vi "Plot Key Down.vi"(7 "Loop data in":T3={"TitleCollapse"=refnum, "MouseDownState"=enum."Idle", "RightClickCache"={"Mod"={"Ctrl"=FALSE, "Shift"=FALSE}, "CoordsStart"={"Horizontal"=0, "Vertical"=0}, "CoordsEnd"={"Horizontal"=0, "Vertical"=0}, "PlotAreaBounds"={"Left"=10, "Top"=10, "Right"=0, "Bottom"=0}, "slice"=[]}, "ZoomCache"={"SuppressedPlots"=[], "LeftAxis"={"NeedsRevert?"=FALSE, "Scale Fit"=0, "Range"={"Minimum"=0.0, "Maximum"=0.0, "Increment"=0.0, "Minor Increment"=0.0, "Start"=0.0}}, "RightAxis"={"NeedsRevert?"=FALSE, "Scale Fit"=0, "Range"={"Minimum"=0.0, "Maximum"=0.0, "Increment"=0.0, "Minor Increment"=0.0, "Start"=0.0}}, "Mod"={"Shift"=FALSE}}, "UpdateTime"=0.0, "keyboard"=refnum, "visible?"=FALSE}, 8 "error in (no error)":errorcluster, 9 "PlatMods":T1, 10 "VKey":T2, 11 "Refs":T14) -> (0 "error out":errorcluster, 3 "Update plot?":bool, 5 "Loop data out":T3={"TitleCollapse"=refnum, "MouseDownState"=enum."Idle", "RightClickCache"={"Mod"={"Ctrl"=FALSE, "Shift"=FALSE}, "CoordsStart"={"Horizontal"=0, "Vertical"=0}, "CoordsEnd"={"Horizontal"=0, "Vertical"=0}, "PlotAreaBounds"={"Left"=10, "Top"=10, "Right"=0, "Bottom"=0}, "slice"=[]}, "ZoomCache"={"SuppressedPlots"=[], "LeftAxis"={"NeedsRevert?"=FALSE, "Scale Fit"=0, "Range"={"Minimum"=0.0, "Maximum"=0.0, "Increment"=0.0, "Minor Increment"=0.0, "Start"=0.0}}, "RightAxis"={"NeedsRevert?"=FALSE, "Scale Fit"=0, "Range"={"Minimum"=0.0, "Maximum"=0.0, "Increment"=0.0, "Minor Increment"=0.0, "Start"=0.0}}, "Mod"={"Shift"=FALSE}}, "UpdateTime"=0.0, "keyboard"=refnum, "visible?"=FALSE})   [LabVIEW 2021, in "RocketPlot.lvlib"]
uses:
  RocketPlot.lvlib
  TypeDefs/Plot UI references.ctl
  Classes/RocketPlotHandle/RocketPlotHandle.lvclass
  <userlib>/bjustice/TipStripOOPanel/Classes/TipPanelHandle/TipPanelHandle.lvclass
  TypeDefs/Plot top row.ctl
  TypeDefs/plot while loop data.ctl
  CollapsePanel/CollapsePanel.lvclass
  TypeDefs/MouseDownState.ctl
  TypeDefs/RightClickCache.ctl
  TypeDefs/RightClickCache PlatMod.ctl
  <vilib>/Utility/miscctls.llb/LVPoint32TypeDef.ctl
  <vilib>/Utility/miscctls.llb/LVRectTypeDef.ctl
  TypeDefs/Slice average.ctl
  TypeDefs/ZoomCache.ctl
  TypeDefs/RangeCache.ctl
  <vilib>/Utility/miscctls.llb/LVRangeTypeDef.ctl
  TypeDefs/ZoomCache PlatMod.ctl
  <vilib>/event_ctls.llb/eventvkey.ctl
  Plot Load maker V2 - scaleread grid colors.vi
  PlatMods to Zoom mods.vi
  Plot scale refnum to LUT name.vi
  Zoom Cache end.vi
  Zoom Cache start.vi
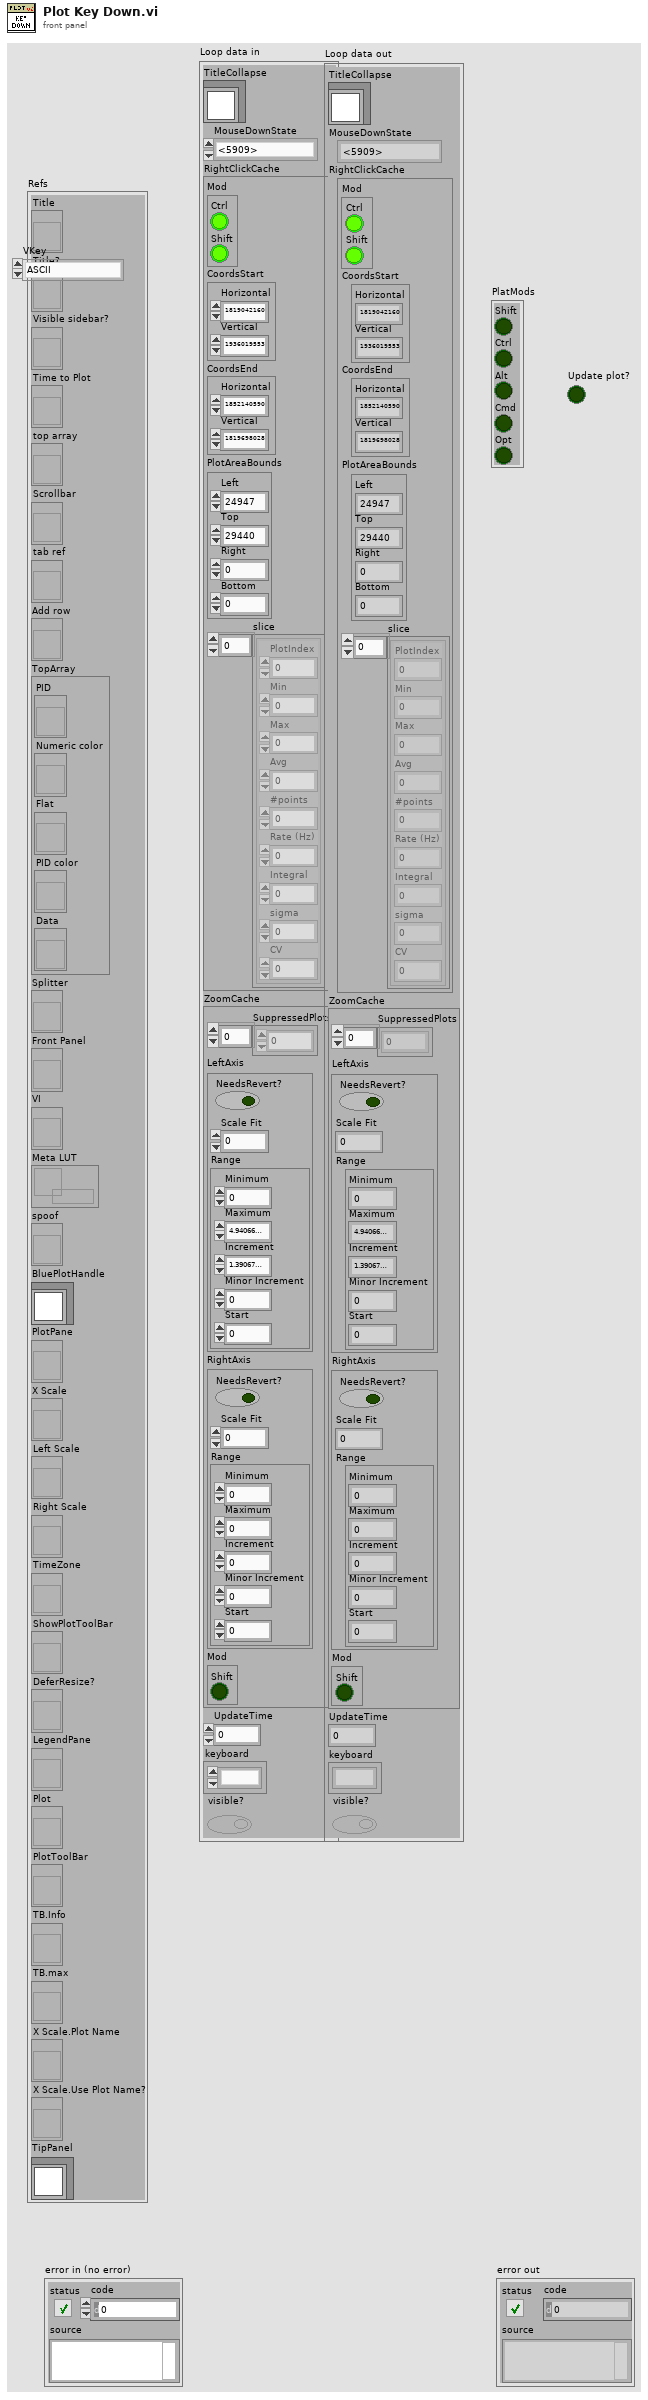
[diagram p1: front panel]
types:
  T1 = cluster{"Shift":bool, "Ctrl":bool, "Alt":bool, "Cmd":bool, "Opt":bool}
  T2 = typedef "eventvkey.ctl" = enum16{"ASCII", "Enter", "Return", "Shift", "Ctrl", "Alt", "Cmd", "Opt", "Caps", "NumLock", "Clear", "Break", "Up", "Down", "Left", "Right", "Insert", "Delete", "Home", "End", "PageUp", "PageDown", "Escape", "Help", "Pause", "ScrollLock", "F1", "F2", "F3", "F4", "F5", "F6", "F7", "F8", "F9", "F10", "F11", "F12", "F13", "F14", "F15", "F16", "F17", "F18", "F19", "F20", "F21", "F22", "F23", "F24", "Play", "VolumeUp", "VolumeDown", "Mute", "Two Byte Char"}
  T3 = typedef "RocketPlot.lvlib/plot while loop data.ctl" = cluster{"TitleCollapse":refnum<class "CollapsePanel.lvclass">, "MouseDownState":T4, "RightClickCache":T5, "ZoomCache":T10, "UpdateTime":dbl, "keyboard":refnum<k1>, "visible?":bool}
  T4 = typedef "RocketPlot.lvlib/MouseDownState.ctl" = enum16{"Idle", "Pan", "Zoom", "Zoom-Post", "RightClick"}
  T5 = typedef "RocketPlot.lvlib/RightClickCache.ctl" = cluster{"Mod":T6, "CoordsStart":T7, "CoordsEnd":T7, "PlotAreaBounds":T8, "slice":T9[]}
  T6 = typedef "RocketPlot.lvlib/RightClickCache PlatMod.ctl" = cluster{"Ctrl":bool, "Shift":bool}
  T7 = typedef "LVPoint32TypeDef.ctl" = cluster{"Horizontal":i32, "Vertical":i32}
  T8 = typedef "LVRectTypeDef.ctl" = cluster{"Left":i16, "Top":i16, "Right":i16, "Bottom":i16}
  T9 = typedef "RocketPlot.lvlib/Slice average.ctl" = cluster{"PlotIndex":i32, "Min":dbl, "Max":dbl, "Avg":dbl, "#points":u32, "Rate (Hz)":dbl, "Integral":dbl, "sigma":dbl, "CV":dbl}
  T10 = typedef "RocketPlot.lvlib/ZoomCache.ctl" = cluster{"SuppressedPlots":i32[], "LeftAxis":T11, "RightAxis":T11, "Mod":T13}
  T11 = typedef "RocketPlot.lvlib/RangeCache.ctl" = cluster{"NeedsRevert?":bool, "Scale Fit":u8, "Range":T12}
  T12 = typedef "LVRangeTypeDef.ctl" = cluster{"Minimum":dbl, "Maximum":dbl, "Increment":dbl, "Minor Increment":dbl, "Start":dbl}
  T13 = typedef "RocketPlot.lvlib/ZoomCache PlatMod.ctl" = cluster{"Shift":bool}
  T14 = typedef "RocketPlot.lvlib/Plot UI references.ctl" = cluster{"Title":refnum<vi>, "Title?":refnum<vi>, "Visible sidebar?":refnum<vi>, "Time to Plot":refnum<vi>, "top array":refnum<vi>, "Scrollbar":refnum<vi>, "tab ref":refnum<vi>, "Add row":refnum<vi>, "TopArray":cluster{"PID":refnum<vi>, "Numeric color":refnum<vi>, "Flat":refnum<vi>, "PID color":refnum<vi>, "Data":refnum<vi>}, "Splitter":refnum<vi>, "Front Panel":refnum<vi>, "VI":refnum<vi>, "Meta LUT":refnum<data-value>, "spoof":refnum<vi>, "BluePlotHandle":refnum<class "RocketPlotHandle.lvclass">, "PlotPane":refnum<vi>, "X Scale":refnum<vi>, "Left Scale":refnum<vi>, "Right Scale":refnum<vi>, "TimeZone":refnum<vi>, "ShowPlotToolBar":refnum<vi>, "DeferResize?":refnum<vi>, "LegendPane":refnum<vi>, "Plot":refnum<vi>, "PlotToolBar":refnum<vi>, "TB.Info":refnum<vi>, "TB.max":refnum<vi>, "X Scale.Plot Name":refnum<vi>, "X Scale.Use Plot Name?":refnum<vi>, "TipPanel":refnum<class "TipPanelHandle.lvclass">}
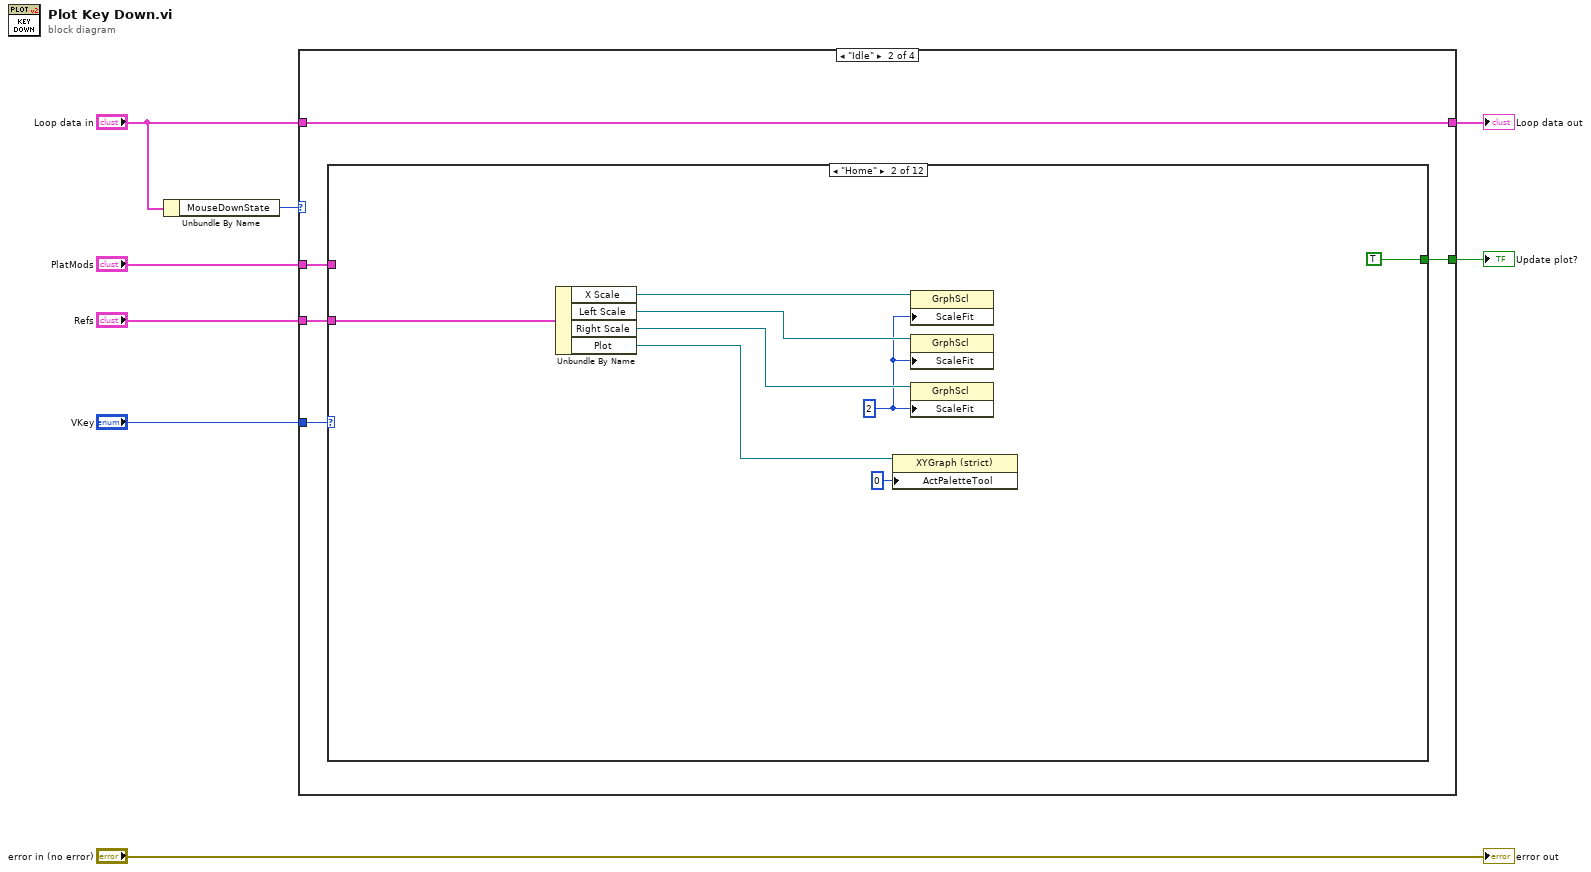
[diagram p0: block diagram]
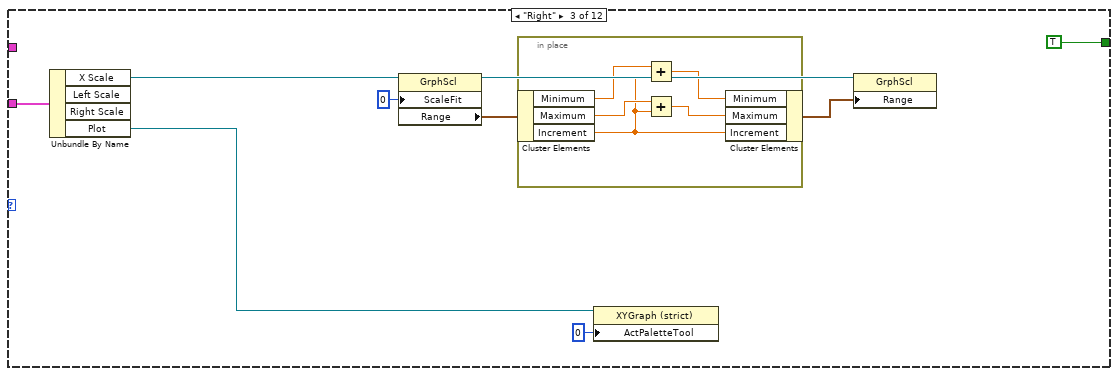
[diagram p4: hidden frame]
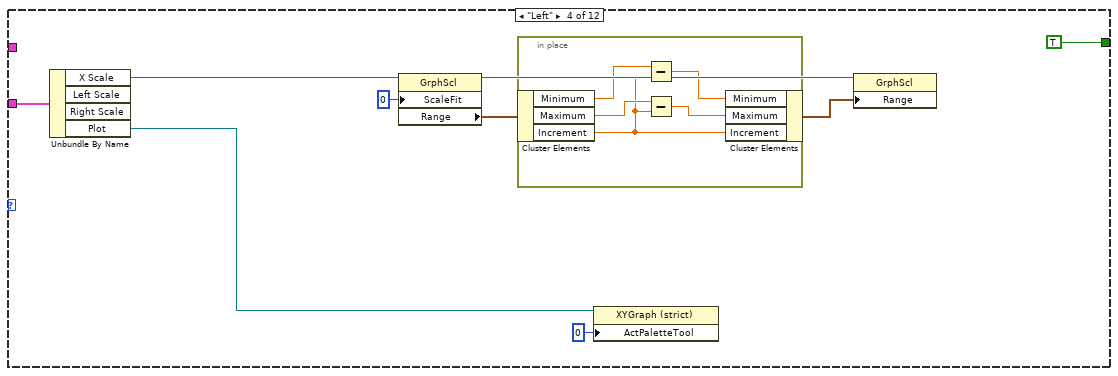
[diagram p5: hidden frame]
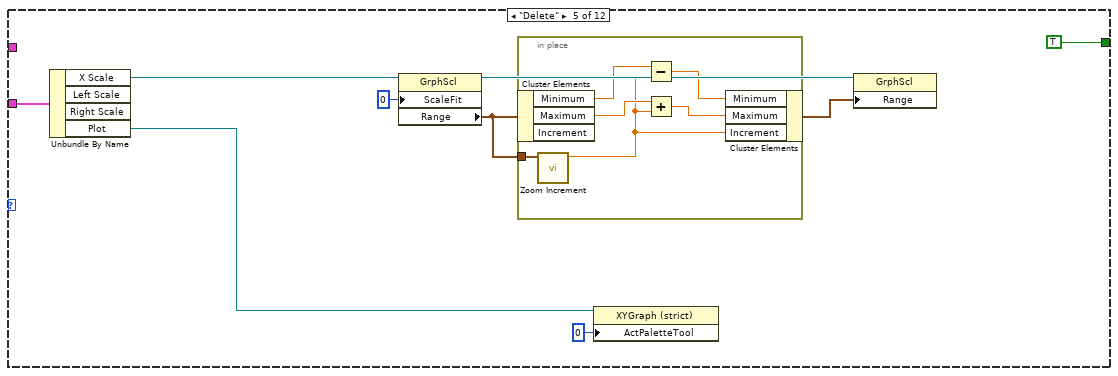
[diagram p6: hidden frame]
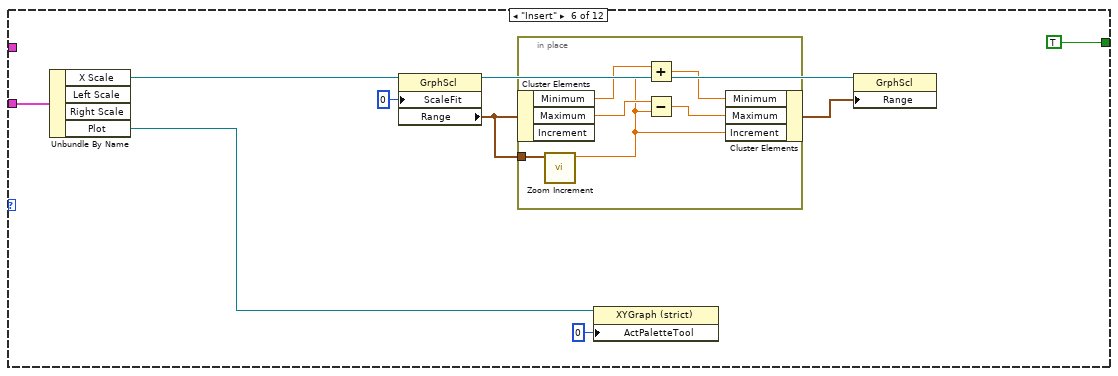
[diagram p7: hidden frame]
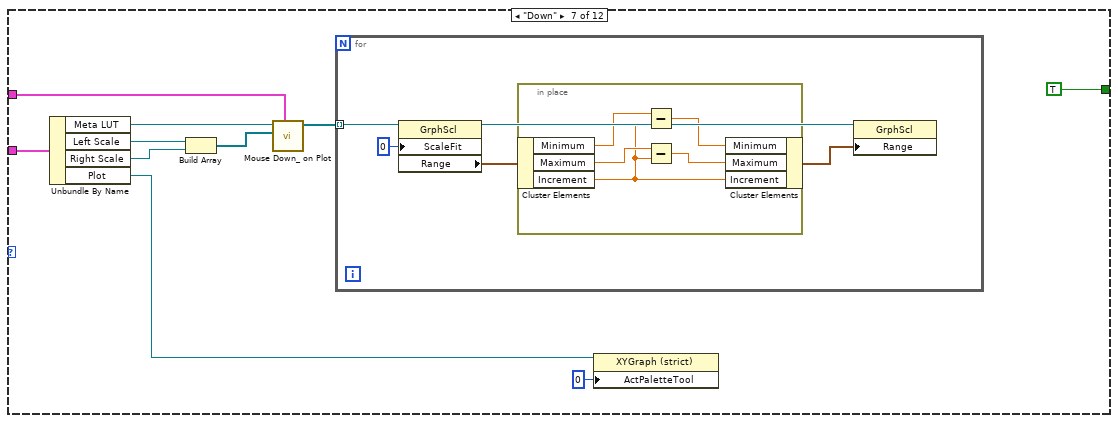
[diagram p8: hidden frame]
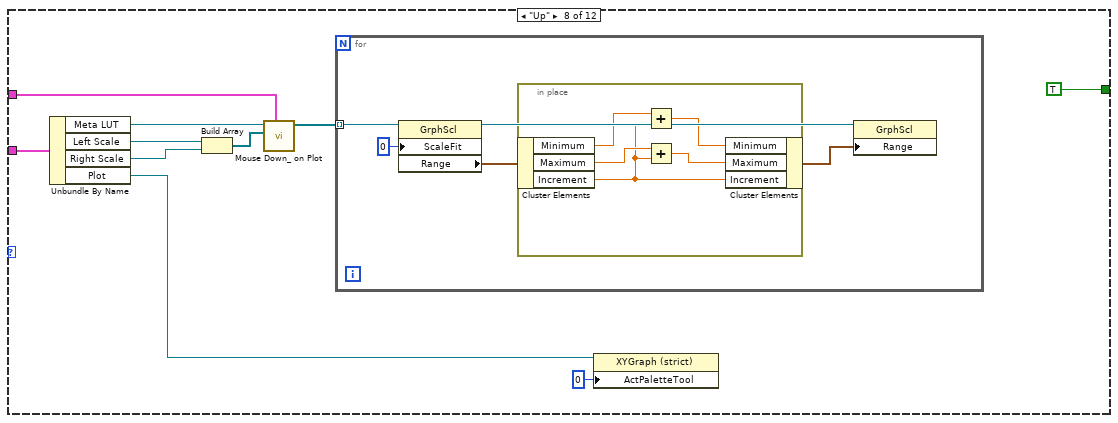
[diagram p9: hidden frame]
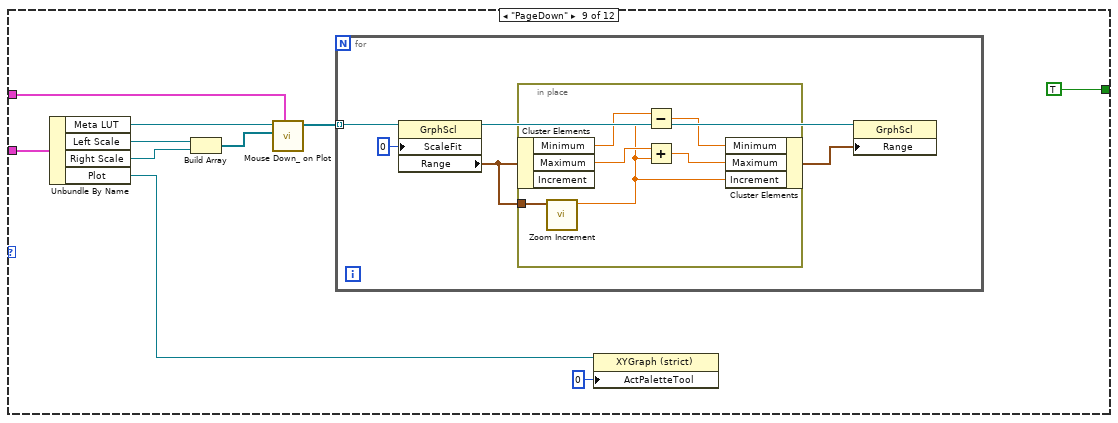
[diagram p10: hidden frame]
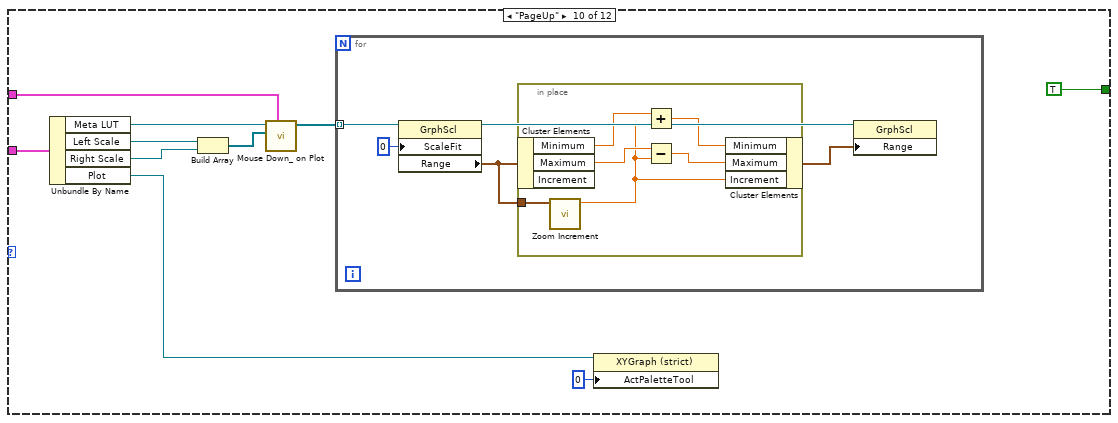
[diagram p11: hidden frame]
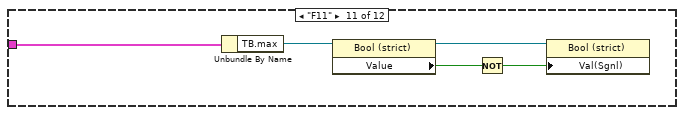
[diagram p12: hidden frame]
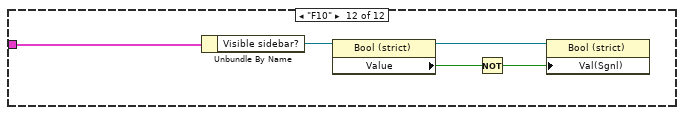
[diagram p13: hidden frame]
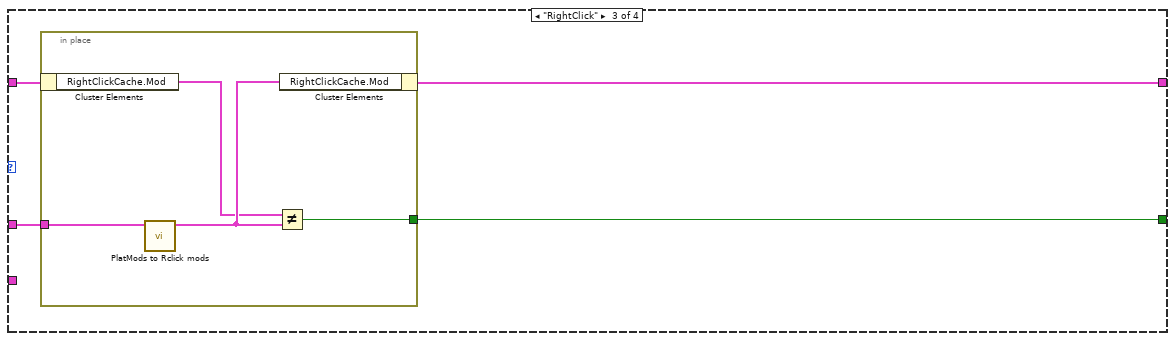
[diagram p14: hidden frame]
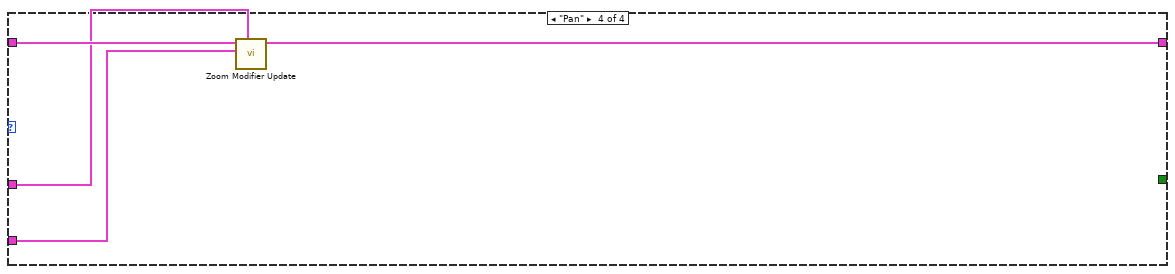
[diagram p15: hidden frame]
diagram:
  n1 = Unbundle By Name("Loop data in") -> ("MouseDownState"=w6:T4)
  n2 = case shown="\"Idle\"" w6 {
    tunnel: "Refs" -> [_ w14 _ w182]
    tunnel: "VKey" -> [_ w13 _ _]
    tunnel: [_ w12 w173 _] -> w4
    tunnel: "PlatMods" -> [_ w11 w175 w183]
    tunnel: "Loop data in" -> [w9 w10 w176 w184]
    tunnel: [w9 w10 w174 w181] -> w1
    frame Default {
    }
    frame "Idle" {
      n3 = case shown="\"Home\"" w13 {
        tunnel: w14 -> [_ w17 w29 w43 w57 w72 w89 w109 w129 w150 w167 w172]
        tunnel: [_ TRUE TRUE TRUE TRUE TRUE TRUE TRUE TRUE TRUE _ _] -> w12
        tunnel: w11 -> [_ _ _ _ _ _ w84 w101 w122 w143 _ _]
        frame Default {
        }
        frame "Home" {
          w18 = u8 2 ("Scale Fit")
          n4 = Unbundle By Name(w17) -> ("X Scale"=w21:refnum<vi>, "Left Scale"=w20:refnum<vi>, "Right Scale"=w19:refnum<vi>, "Plot"=w16:refnum<vi>)
          n5 = property class="XYGraph (strict)"(reference=w16, "ActPaletteTool"=0 ("Palette:Active Tool")) -> ()  [unwired: 1 in, 2 out]
          n6 = property class="GrphScl"(reference=w21, "ScaleFit"=w18) -> ()  [unwired: 1 in, 2 out]
          n7 = property class="GrphScl"(reference=w20, "ScaleFit"=w18) -> ()  [unwired: 1 in, 2 out]
          n8 = property class="GrphScl"(reference=w19, "ScaleFit"=w18) -> ()  [unwired: 1 in, 2 out]
        }
        frame "Right" {
          n9 = Unbundle By Name(w29) -> ("X Scale"=w30:refnum<vi>, "Plot"=w28:refnum<vi>)  [unwired: 2 out]
          n10 = property class="GrphScl"(reference=w30, "ScaleFit"=u8 0 ("Scale Fit")) -> (reference out=w26:refnum<vi>, "Range"=w25:T12)  [unwired: 1 in, 1 out]
          n11 = in-place {
            n12 = in-place-cluster #1(w25) -> ("Minimum"=w36:dbl, "Maximum"=w34:dbl, "Increment"=w32:dbl)
            n13 = Add(x=w36, y=w32) -> (x+y=w35:dbl)
            n14 = Add(x=w34, y=w32) -> (x+y=w33:dbl)
            n15 = in-place-cluster #1("Minimum"=w35, "Maximum"=w33, "Increment"=w32) -> (w24:T12)
          }
          n16 = property class="XYGraph (strict)"(reference=w28, "ActPaletteTool"=0 ("Palette:Active Tool")) -> ()  [unwired: 1 in, 2 out]
          n17 = property class="GrphScl"(reference=w26, "Range"=w24) -> ()  [unwired: 1 in, 2 out]
        }
        frame "Left" {
          n18 = Unbundle By Name(w43) -> ("X Scale"=w44:refnum<vi>, "Plot"=w42:refnum<vi>)  [unwired: 2 out]
          n19 = property class="GrphScl"(reference=w44, "ScaleFit"=u8 0 ("Scale Fit")) -> (reference out=w40:refnum<vi>, "Range"=w39:T12)  [unwired: 1 in, 1 out]
          n20 = in-place {
            n21 = in-place-cluster #2(w39) -> ("Minimum"=w50:dbl, "Maximum"=w48:dbl, "Increment"=w46:dbl)
            n22 = Subtract(x=w50, y=w46) -> (x-y=w49:dbl)
            n23 = Subtract(x=w48, y=w46) -> (x-y=w47:dbl)
            n24 = in-place-cluster #2("Minimum"=w49, "Maximum"=w47, "Increment"=w46) -> (w38:T12)
          }
          n25 = property class="XYGraph (strict)"(reference=w42, "ActPaletteTool"=0 ("Palette:Active Tool")) -> ()  [unwired: 1 in, 2 out]
          n26 = property class="GrphScl"(reference=w40, "Range"=w38) -> ()  [unwired: 1 in, 2 out]
        }
        frame "Delete" {
          n27 = Unbundle By Name(w57) -> ("X Scale"=w58:refnum<vi>, "Plot"=w56:refnum<vi>)  [unwired: 2 out]
          n28 = property class="GrphScl"(reference=w58, "ScaleFit"=u8 0 ("Scale Fit")) -> (reference out=w54:refnum<vi>, "Range"=w51:T12)  [unwired: 1 in, 1 out]
          n29 = in-place {
            in-place-border: w51 -> [w61]
            n30 = in-place-cluster #3(w51) -> ("Minimum"=w65:dbl, "Maximum"=w63:dbl)  [unwired: 1 out]
            n31 = call "Zoom Increment.vi"("Range"=w61) -> ("Increment"=w60:dbl)  [unwired: 10 in]
            n32 = Subtract(x=w65, y=w60) -> (x-y=w64:dbl)
            n33 = Add(x=w63, y=w60) -> (x+y=w62:dbl)
            n34 = in-place-cluster #3("Minimum"=w64, "Maximum"=w62, "Increment"=w60) -> (w53:T12)
          }
          n35 = property class="XYGraph (strict)"(reference=w56, "ActPaletteTool"=0 ("Palette:Active Tool")) -> ()  [unwired: 1 in, 2 out]
          n36 = property class="GrphScl"(reference=w54, "Range"=w53) -> ()  [unwired: 1 in, 2 out]
        }
        frame "Insert" {
          n37 = Unbundle By Name(w72) -> ("X Scale"=w73:refnum<vi>, "Plot"=w71:refnum<vi>)  [unwired: 2 out]
          n38 = property class="GrphScl"(reference=w73, "ScaleFit"=u8 0 ("Scale Fit")) -> (reference out=w69:refnum<vi>, "Range"=w66:T12)  [unwired: 1 in, 1 out]
          n39 = in-place {
            in-place-border: w66 -> [w76]
            n40 = in-place-cluster #4(w66) -> ("Minimum"=w80:dbl, "Maximum"=w78:dbl)  [unwired: 1 out]
            n41 = call "Zoom Increment.vi"("Range"=w76) -> ("Increment"=w75:dbl)  [unwired: 10 in]
            n42 = Add(x=w80, y=w75) -> (x+y=w79:dbl)
            n43 = Subtract(x=w78, y=w75) -> (x-y=w77:dbl)
            n44 = in-place-cluster #4("Minimum"=w79, "Maximum"=w77, "Increment"=w75) -> (w68:T12)
          }
          n45 = property class="XYGraph (strict)"(reference=w71, "ActPaletteTool"=0 ("Palette:Active Tool")) -> ()  [unwired: 1 in, 2 out]
          n46 = property class="GrphScl"(reference=w69, "Range"=w68) -> ()  [unwired: 1 in, 2 out]
        }
        frame "Down" {
          n47 = Unbundle By Name(w89) -> ("Meta LUT"=w83:refnum<data-value>, "Left Scale"=w86:refnum<vi>, "Right Scale"=w85:refnum<vi>, "Plot"=w88:refnum<vi>)
          n48 = Build Array(w86, w85) -> (w82:refnum<vi>[])
          n49 = call "Mouse Down_ on Plot.vi"("PlatMods"=w84, "Y axes"=w82, "Meta LUT"=w83) -> ("axes to scale"=w81:refnum<vi>[])  [unwired: 6 in, 2 out]
          n50 = for {
            tunnel: w81 -> [w91] mode=indexing
            n51 = property class="GrphScl"(reference=w91, "ScaleFit"=u8 0 ("Scale Fit")) -> (reference out=w94:refnum<vi>, "Range"=w93:T12)  [unwired: 1 in, 1 out]
            n52 = in-place {
              n53 = in-place-cluster #5(w93) -> ("Minimum"=w100:dbl, "Maximum"=w98:dbl, "Increment"=w96:dbl)
              n54 = Subtract(x=w100, y=w96) -> (x-y=w99:dbl)
              n55 = Subtract(x=w98, y=w96) -> (x-y=w97:dbl)
              n56 = in-place-cluster #5("Minimum"=w99, "Maximum"=w97, "Increment"=w96) -> (w92:T12)
            }
            n57 = property class="GrphScl"(reference=w94, "Range"=w92) -> ()  [unwired: 1 in, 2 out]
          }
          n58 = property class="XYGraph (strict)"(reference=w88, "ActPaletteTool"=0 ("Palette:Active Tool")) -> ()  [unwired: 1 in, 2 out]
        }
        frame "Up" {
          n59 = Unbundle By Name(w109) -> ("Meta LUT"=w104:refnum<data-value>, "Left Scale"=w106:refnum<vi>, "Right Scale"=w105:refnum<vi>, "Plot"=w108:refnum<vi>)
          n60 = Build Array(w106, w105) -> (w102:refnum<vi>[])
          n61 = call "Mouse Down_ on Plot.vi"("PlatMods"=w101, "Y axes"=w102, "Meta LUT"=w104) -> ("axes to scale"=w103:refnum<vi>[])  [unwired: 6 in, 2 out]
          n62 = for {
            tunnel: w103 -> [w112] mode=indexing
            n63 = property class="GrphScl"(reference=w112, "ScaleFit"=u8 0 ("Scale Fit")) -> (reference out=w114:refnum<vi>, "Range"=w111:T12)  [unwired: 1 in, 1 out]
            n64 = in-place {
              n65 = in-place-cluster #6(w111) -> ("Minimum"=w120:dbl, "Maximum"=w118:dbl, "Increment"=w116:dbl)
              n66 = Add(x=w120, y=w116) -> (x+y=w119:dbl)
              n67 = Add(x=w118, y=w116) -> (x+y=w117:dbl)
              n68 = in-place-cluster #6("Minimum"=w119, "Maximum"=w117, "Increment"=w116) -> (w113:T12)
            }
            n69 = property class="GrphScl"(reference=w114, "Range"=w113) -> ()  [unwired: 1 in, 2 out]
          }
          n70 = property class="XYGraph (strict)"(reference=w108, "ActPaletteTool"=0 ("Palette:Active Tool")) -> ()  [unwired: 1 in, 2 out]
        }
        frame "PageDown" {
          n71 = Unbundle By Name(w129) -> ("Meta LUT"=w123:refnum<data-value>, "Left Scale"=w126:refnum<vi>, "Right Scale"=w125:refnum<vi>, "Plot"=w128:refnum<vi>)
          n72 = Build Array(w126, w125) -> (w124:refnum<vi>[])
          n73 = call "Mouse Down_ on Plot.vi"("PlatMods"=w122, "Y axes"=w124, "Meta LUT"=w123) -> ("axes to scale"=w121:refnum<vi>[])  [unwired: 6 in, 2 out]
          n74 = for {
            tunnel: w121 -> [w132] mode=indexing
            n75 = property class="GrphScl"(reference=w132, "ScaleFit"=u8 0 ("Scale Fit")) -> (reference out=w134:refnum<vi>, "Range"=w131:T12)  [unwired: 1 in, 1 out]
            n76 = in-place {
              in-place-border: w131 -> [w137]
              n77 = in-place-cluster #7(w131) -> ("Minimum"=w141:dbl, "Maximum"=w139:dbl)  [unwired: 1 out]
              n78 = call "Zoom Increment.vi"("Range"=w137) -> ("Increment"=w136:dbl)  [unwired: 10 in]
              n79 = Subtract(x=w141, y=w136) -> (x-y=w140:dbl)
              n80 = Add(x=w139, y=w136) -> (x+y=w138:dbl)
              n81 = in-place-cluster #7("Minimum"=w140, "Maximum"=w138, "Increment"=w136) -> (w133:T12)
            }
            n82 = property class="GrphScl"(reference=w134, "Range"=w133) -> ()  [unwired: 1 in, 2 out]
          }
          n83 = property class="XYGraph (strict)"(reference=w128, "ActPaletteTool"=0 ("Palette:Active Tool")) -> ()  [unwired: 1 in, 2 out]
        }
        frame "PageUp" {
          n84 = Unbundle By Name(w150) -> ("Meta LUT"=w144:refnum<data-value>, "Left Scale"=w147:refnum<vi>, "Right Scale"=w146:refnum<vi>, "Plot"=w149:refnum<vi>)
          n85 = Build Array(w147, w146) -> (w145:refnum<vi>[])
          n86 = call "Mouse Down_ on Plot.vi"("PlatMods"=w143, "Y axes"=w145, "Meta LUT"=w144) -> ("axes to scale"=w142:refnum<vi>[])  [unwired: 6 in, 2 out]
          n87 = for {
            tunnel: w142 -> [w153] mode=indexing
            n88 = property class="GrphScl"(reference=w153, "ScaleFit"=u8 0 ("Scale Fit")) -> (reference out=w155:refnum<vi>, "Range"=w152:T12)  [unwired: 1 in, 1 out]
            n89 = in-place {
              in-place-border: w152 -> [w158]
              n90 = in-place-cluster #8(w152) -> ("Minimum"=w162:dbl, "Maximum"=w160:dbl)  [unwired: 1 out]
              n91 = call "Zoom Increment.vi"("Range"=w158) -> ("Increment"=w157:dbl)  [unwired: 10 in]
              n92 = Add(x=w162, y=w157) -> (x+y=w161:dbl)
              n93 = Subtract(x=w160, y=w157) -> (x-y=w159:dbl)
              n94 = in-place-cluster #8("Minimum"=w161, "Maximum"=w159, "Increment"=w157) -> (w154:T12)
            }
            n95 = property class="GrphScl"(reference=w155, "Range"=w154) -> ()  [unwired: 1 in, 2 out]
          }
          n96 = property class="XYGraph (strict)"(reference=w149, "ActPaletteTool"=0 ("Palette:Active Tool")) -> ()  [unwired: 1 in, 2 out]
        }
        frame "F11" {
          n97 = Unbundle By Name(w167) -> ("TB.max"=w166:refnum<vi>)
          n98 = property class="Bool (strict)"(reference=w166) -> (reference out=w164:refnum<vi>, "Value"=w165:bool)  [unwired: 1 in, 1 out]
          n99 = Not(x=w165) -> (.not. x?=w163:bool)
          n100 = property class="Bool (strict)"(reference=w164, "Val(Sgnl)"=w163) -> ()  [unwired: 1 in, 2 out]
        }
        frame "F10" {
          n101 = Unbundle By Name(w172) -> ("Visible sidebar?"=w171:refnum<vi>)
          n102 = property class="Bool (strict)"(reference=w171) -> (reference out=w169:refnum<vi>, "Value"=w170:bool)  [unwired: 1 in, 1 out]
          n103 = Not(x=w170) -> (.not. x?=w168:bool)
          n104 = property class="Bool (strict)"(reference=w169, "Val(Sgnl)"=w168) -> ()  [unwired: 1 in, 2 out]
        }
      }
    }
    frame "RightClick" {
      n105 = in-place {
        in-place-border: w175 -> [w180]
        in-place-border: [w177] -> w173
        n106 = in-place-cluster #9(w176) -> ("RightClickCache.Mod"=w178:T6)
        n107 = call "PlatMods to Rclick mods.vi"("PlatMods"=w180) -> ("Rclick mods"=w179:T6)  [unwired: 10 in]
        n108 = Not Equal?(x=w178, y=w179) -> (x != y?=w177:bool)
        n109 = in-place-cluster #9("RightClickCache.Mod"=w179) -> (w174:T3)
      }
    }
    frame "Pan" {
      n110 = call "Zoom Modifier Update.vi"("PlatMods"=w183, "Refs"=w182, "Loop data in"=w184) -> ("Loop data out"=w181:T3)  [unwired: 7 in, 1 out]
    }
  }
  "Loop data out" <- w1
  "Update plot?" <- w4
  "error out" <- "error in (no error)"
